vi "Get SMO Public API Documentation.vi"(8 "error in (no error)":errorcluster, 11 "Instrument in":refnum<class "Instrument.lvclass">) -> (0 "error out":errorcluster, 2 "<JSON> API documentation":string, 3 "Instrument out":refnum<class "Instrument.lvclass">)   [LabVIEW 2019, in "Instrument.lvclass"]
doc: "Override this VI to return a list of commands supported by your Instrument"
uses:
  Instrument.lvclass
  Typedefs/Instrument.Commands--Enum.ctl
  Help/Help.lvclass
  Help/Help.lvclass/Help.ctl
  Typedefs/Instrument.API_Help--Map.ctl
  Typedefs/Instrument.API_Help--Cluster.ctl
  Typedefs/Instrument.API_Help.Param--Cluster.ctl
  ad9b2bd1-4baa-4139-994d-e1b6d0ed2716.vi
  662017c9-57ff-4788-a91f-1902fc938222.vi
  c00cddf8-8320-4c92-b56e-c453e6deb51d.vi
  662017c9-57ff-4788-a91f-1902fc938222.vi/8df63497-2dec-42cd-aa00-23db4ff10e9d.vi
  <vilib>/Utility/Data Type/Get Numeric Information.vi
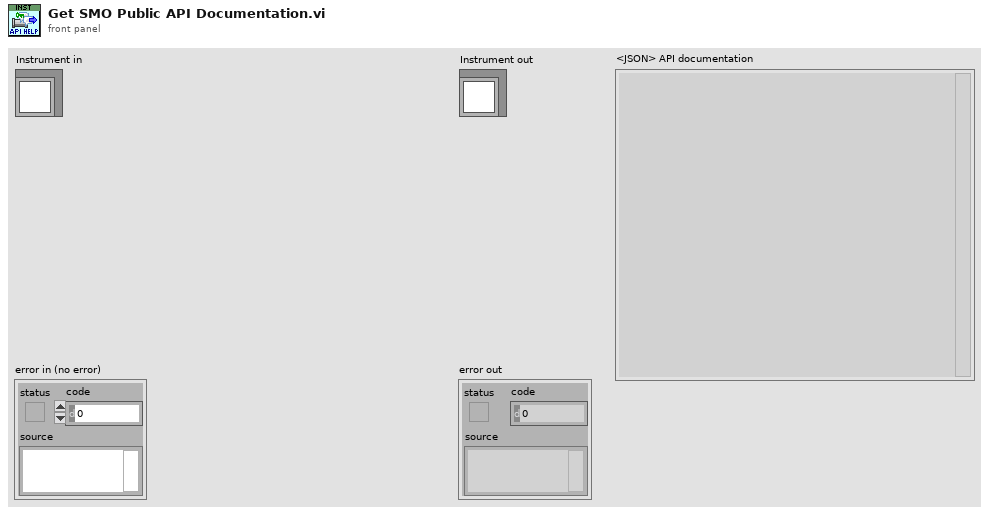
[diagram p1: front panel]
types:
  T1 = typedef "Instrument.lvclass/Instrument.Commands--Enum.ctl" = enum16{"ACK", "HELP", "setConfiguration", "setLogData", "getAll", "getAllData"}
  T2 = typedef "Instrument.lvclass/Instrument.API_Help--Map.ctl" = map{string, T3}
  T3 = typedef "Instrument.lvclass/Instrument.API_Help--Cluster.ctl" = cluster{"command":string, "description":string, "parameters":map{string, T4}, "jsonrpc_example":string}
  T4 = typedef "Instrument.lvclass/Instrument.API_Help.Param--Cluster.ctl" = cluster{"parameter_name":string, "description":string, "min_value":variant, "max_value":variant, "units":string}
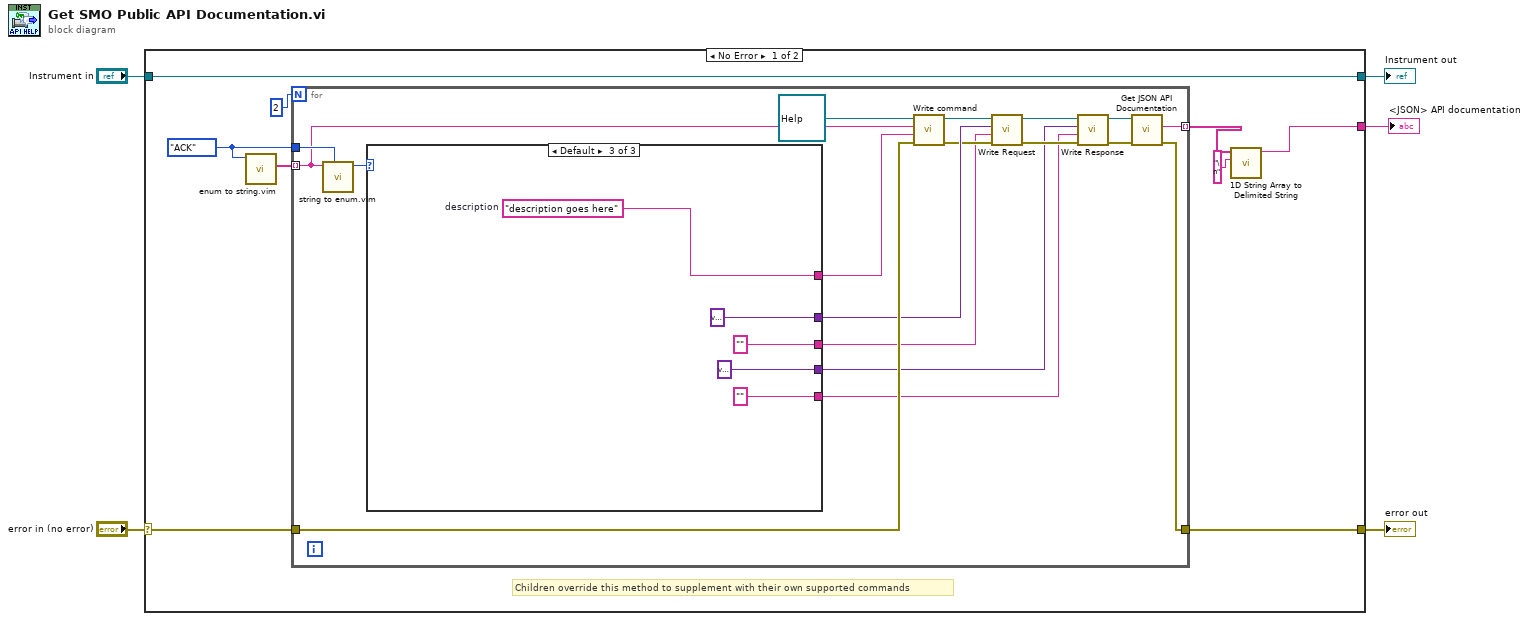
[diagram p0: block diagram]
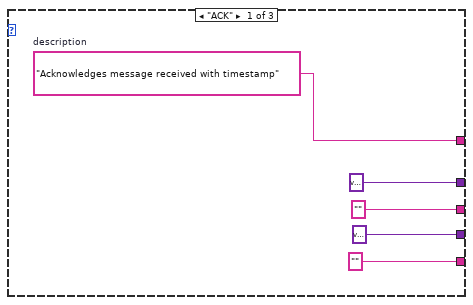
[diagram p2: hidden frame]
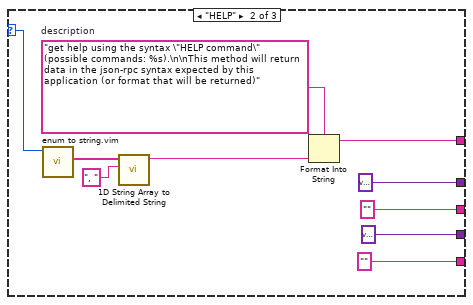
[diagram p3: hidden frame]
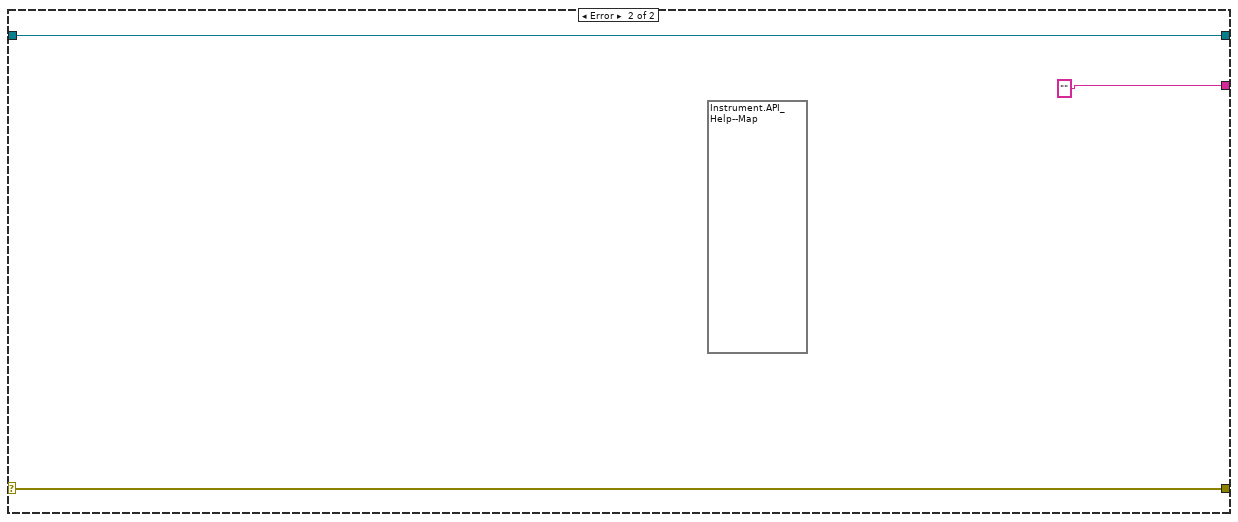
[diagram p4: hidden frame]
diagram:
  n1 = case shown="No Error" "error in (no error)" {
    selector: "error in (no error)" -> [w11 w55]
    tunnel: [w10 w55] -> w4
    tunnel: [w12 w54] -> w2
    tunnel: "Instrument in" -> [w12 w54]
    tunnel: [w7 "" ("<JSON> API documentation")] -> w1
    frame No Error {
      w13 = Instrument.Commands--Enum."ACK" ("Commands")
      # "Children override this method to supplement with their own supported commands"
      n2 = call "enum to string.vim"("enum in"=w13) -> ("strings out"=w14:string[])  [unwired: 9 in, 1 out]
      n3 = for {
        N: 2 -> [_]
        tunnel: w14 -> [w27] mode=indexing
        tunnel: w13 -> [w31]
        tunnel: w11 -> [w29]
        tunnel: [w28] -> w10
        tunnel: [w30] -> w8 mode=indexing
        n4 = call "string to enum.vim"("enum type"=w31, "string in"=w27) -> ("enum out"=w32:T1)  [unwired: 9 in]
        n5 = case shown="Default" w32 {
          selector: w32 -> [_ w47 _]
          tunnel: [w37 w42 w52] -> w24
          tunnel: ["" ("<JSON> response documentation") "" ("<JSON> response documentation") "" ("<JSON> response documentation")] -> w15
          tunnel: [variant ("response cluster") variant ("response cluster") variant ("response cluster")] -> w16
          tunnel: ["" ("<JSON> request documentation") "" ("<JSON> request documentation") "" ("<JSON> request documentation")] -> w21
          tunnel: [variant ("request cluster") variant ("request cluster") variant ("request cluster")] -> w26
          frame "ACK" {
            w37 = "Acknowledges message received with timestamp"  # description
          }
          frame "HELP" {
            w43 = "get help using the syntax \"HELP command\" (possible commands: %s).\n\nThis method will return data in the json-rpc syntax expected by this application (or format that will be returned)"  # description
            n6 = call "enum to string.vim"("enum in"=w47) -> ("strings out"=w46:string[])  [unwired: 9 in, 1 out]
            n7 = call <vilib>:"1D String Array to Delimited String.vi"("delimiter"=", ", "string array"=w46) -> ("delimited string"=w45:string)  [unwired: 9 in]
            n8 = Format Into String(format string=w43, w45) -> (resulting string=w42:string)  [unwired: 2 in, 1 out]
          }
          frame Default {
            w52 = "description goes here"  # description
          }
        }
        n9 = call "Write command.vi"("error in (no error)"=w29, "command description"=w24, "command"=w27, "Help in"=refnum<class "Help.lvclass"> refnum) -> ("error out"=w22:errorcluster, "Help out"=w23:refnum<class "Help.lvclass">)  [unwired: 6 in]
        n10 = call "Write Request.vi"("error in (no error)"=w22, "<JSON> request documentation"=w21, "request cluster"=w26, "Help in"=w23) -> ("error out"=w19:errorcluster, "Help out"=w20:refnum<class "Help.lvclass">)  [unwired: 6 in]
        n11 = call "Write Response.vi"("error in (no error)"=w19, "<JSON> response documentation"=w15, "response cluster"=w16, "Help in"=w20) -> ("error out"=w17:errorcluster, "Help out"=w18:refnum<class "Help.lvclass">)  [unwired: 6 in]
        n12 = call "Get JSON API Documentation.vi"("error in (no error)"=w17, "Help"=w18) -> ("error out"=w28:errorcluster, "<JSON> API documentation"=w30:string)  [unwired: 7 in, 1 out]
      }
      n13 = call <vilib>:"1D String Array to Delimited String.vi"("delimiter"="\n", "string array"=w8) -> ("delimited string"=w7:string)  [unwired: 9 in]
    }
    frame Error {
      (unwired) T2 {} ("documentation")
    }
  }
  "error out" <- w4
  "Instrument out" <- w2
  "<JSON> API documentation" <- w1
